vi "Linear Transform.vi"(11 "Right Motor Value":dbl) -> (3 "Transformed":dbl)   [LabVIEW 2019]
panel:
  in  "b":dbl
  in  "m":dbl
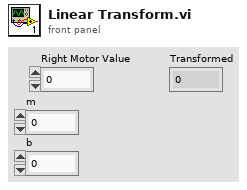
[diagram p1: front panel]
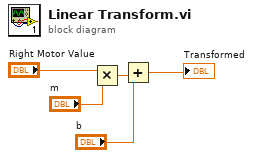
[diagram p0: block diagram]
diagram:
  n1 = Multiply(x="Right Motor Value", y="m") -> (x*y=w3:dbl)
  n2 = Add(x="b", y=w3) -> (x+y=→"Transformed":dbl)
